vi "ListDatabases.vi"(8 "error in (no error)":errorcluster, 11 "MongoDB-Client in":refnum<class "MongoDB-Client.lvclass">) -> (0 "error out":errorcluster, 2 "ListDatabases":string[](array[string]), 3 "MongoDB-Client out":refnum<class "MongoDB-Client.lvclass">)   [LabVIEW 2016, in "MongoDB-Client.lvlib" / "MongoDB-Client.lvclass"]
uses:
  MongoDB-Client.lvclass
  D:/Users/blume/Desktop/LV/MongoDB-Driver/MLV DLLs/MongoLabVIEW.dll
  LV/MongoDB-Driver/MLV DLLs/MongoLabVIEW.dll
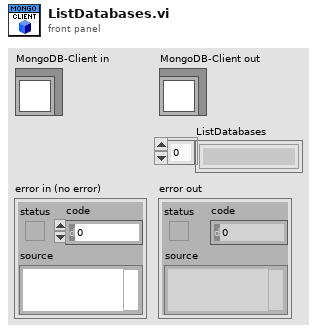
[diagram p1: front panel]
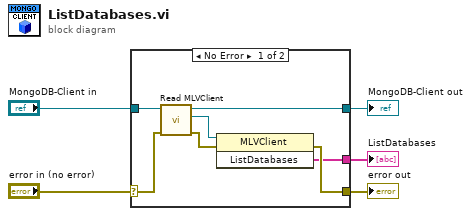
[diagram p0: block diagram]
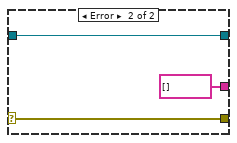
[diagram p2: hidden frame]
diagram:
  n1 = case shown="No Error" "error in (no error)" {
    selector: "error in (no error)" -> [w10 w15]
    tunnel: [w7 w15] -> w4
    tunnel: [w11 w14] -> w2
    tunnel: "MongoDB-Client in" -> [w12 w14]
    tunnel: [w6 string[] [] ("ListDatabases")] -> w1
    frame No Error {
      n2 = call "Read MLVClient.vi"("error in (no error)"=w10, "MongoDB-Client in"=w12) -> ("error out"=w8:errorcluster, "MLVClient"=w9:refnum<k24>, "MongoDB-Client out"=w11:refnum<class "MongoDB-Client.lvclass">)  [unwired: 7 in]
      n3 = invoke class="MLVClient" method="ListDatabases"(reference=w9, error in=w8) -> (error out=w7:errorcluster, "ListDatabases"=w6:string[])  [unwired: 1 in, 1 out]
    }
    frame Error {
    }
  }
  "error out" <- w4
  "MongoDB-Client out" <- w2
  "ListDatabases" <- w1
